vi "Config - resolve.vi"(8 "error in (no error)":errorcluster) -> (0 "error out":errorcluster)   [LabVIEW 2026, in "Tests.lvlib"]
doc: "Unit test (Caraya) for launch-config resolution.\nWith no config path the effective config equals the baseline inputs; a defined-but-missing path returns a non-fatal warning and falls back to the baseline; a present-but-invalid file (unparseable or schema-invalid) fails launch with no fallback.\nThe no-path and missing-path cases need no file; the invalid-file cases use a temp-root fixture that writes a malformed and a schema-invalid JSON file. Each expected error is captured and cleared per case.\n\nImplements LMBR-T-020, T-022, T-023 -> SRS-044, SRS-047, SRS-048. Assert-level IDs: Test-ID-Assert-Checklist.md."
uses:
  Tests.lvlib
  <vilib>/addons/_JKI Toolkits/Caraya/classes/Test/Test.lvclass
  <vilib>/addons/_JKI Toolkits/Caraya/classes/Assert/Assert.lvclass
  <vilib>/addons/_JKI Toolkits/Caraya/classes/Assert/Assert Equal Value_Variant.vi
  src/Lumberjack.lvlib
  src/TypeDefs/Severity.ctl
  src/TypeDefs/FilterMode.ctl
  src/TypeDefs/Filter.ctl
  src/TypeDefs/DropPolicy.ctl
  src/TypeDefs/AppenderConfig.ctl
  src/TypeDefs/FileConfig.ctl
  src/TypeDefs/FileAppenderConfig.ctl
  <vilib>/addons/_JKI Toolkits/Caraya/classes/Assert/Assert Error.vi
  <vilib>/addons/_JKI Toolkits/Caraya/classes/Assert/Assert False.vi
  <vilib>/addons/_JKI Toolkits/Caraya/classes/Assert/Assert True.vi
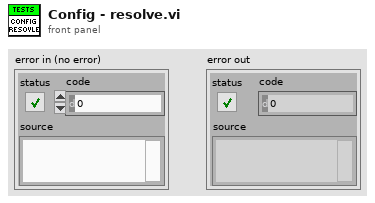
[diagram p1: front panel]
types:
  T1 = typedef "Lumberjack.lvlib/Severity.ctl" = enum16{"OFF", "FATAL", "ERROR", "WARN", "INFO", "DEBUG", "TRACE", "ALL"}
  T2 = typedef "Lumberjack.lvlib/FileAppenderConfig.ctl" = cluster{"common":T3, "file":T7}
  T3 = typedef "Lumberjack.lvlib/AppenderConfig.ctl" = cluster{"id":string, "threshold":T1, "filter":T4, "queueBound":i32, "dropPolicy":T6, "useUTC":bool}
  T4 = typedef "Lumberjack.lvlib/Filter.ctl" = cluster{"mode":T5, "levelMin":T1, "levelMax":T1, "tagPrefix":string}
  T5 = typedef "Lumberjack.lvlib/FilterMode.ctl" = enum16{"Mirror", "Routed"}
  T6 = typedef "Lumberjack.lvlib/DropPolicy.ctl" = enum16{"DropOldest", "DropNewest", "LevelAware"}
  T7 = typedef "Lumberjack.lvlib/FileConfig.ctl" = cluster{"rootFolder":path, "maxFileSize":i64, "maxFileCount":i32, "baseName":string, "extension":string, "delimiter":string, "calendarFolderTree":bool}
  T8 = typedef "Lumberjack.lvlib/LumberjackConfig.ctl" = cluster{"schemaVersion":string, "globalThreshold":T1, "defaultFileAppender":T2}
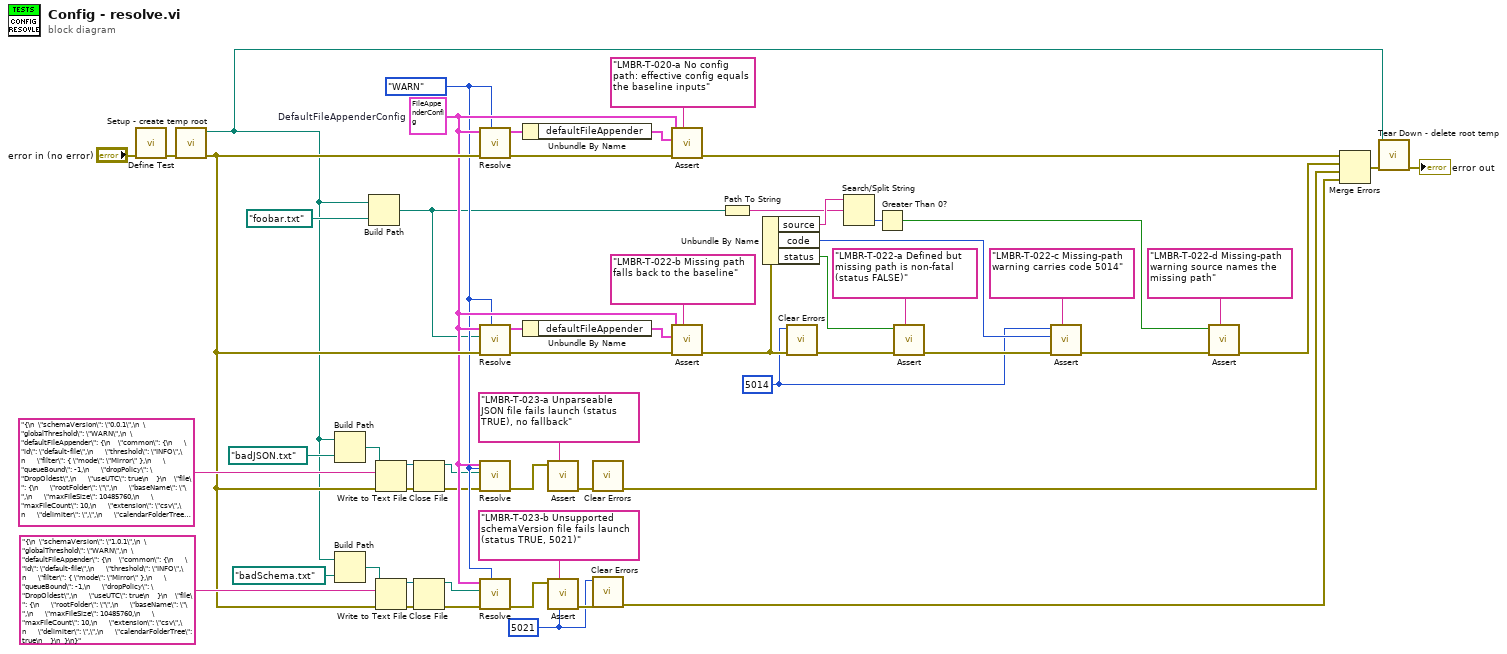
[diagram p0: block diagram]
diagram:
  w12 = 5014 ("error code (1)")
  w32 = 5021 ("error code (1)")
  w36 = Severity."WARN" ("GlobalThreshold")
  w37 = T2 {"common"={"id"="cfg-test", "threshold"=enum."ERROR", "filter"={"mode"=enum."Mirror", "levelMin"=enum."INFO", "levelMax"=enum."INFO", "tagPrefix"=""}, "queueBound"=250, "dropPolicy"=enum."DropNewest", "useUTC"=FALSE}, "file"={"rootFolder"=path "c:/Logs/cfgtest", "maxFileSize"=2097152, "maxFileCount"=7, "baseName"="cfg", "extension"="log", "delimiter"=";", "calendarFolderTree"=FALSE}}  # DefaultFileAppenderConfig
  n1 = call <vilib>:"Define Test.vi"("error in (no error)"="error in (no error)") -> ("error out"=w46:errorcluster)  [unwired: 9 in, 1 out]
  n2 = call "Setup - create temp root.vi"("error in (no error)"=w46) -> ("error out"=w38:errorcluster, "tempRoot"=w26:path)  [unwired: 9 in]
  n3 = Build Path(base path=w26, name or relative path=path "badJSON.txt") -> (appended path=w43:path)
  n4 = Build Path(base path=w26, name or relative path=path "badSchema.txt") -> (appended path=w39:path)
  n5 = Build Path(base path=w26, name or relative path=path "foobar.txt") -> (appended path=w20:path)
  n6 = Write to Text File(file (use dialog)=w43, text="{\n  \"schemaVersion\": \"0.0.1\",\n  \"globalThreshold\": \"WARN\",\n  \"defaultFileAppender\": {\n    \"common\": {\n      \"id\": \"default-file\",\n      \"threshold\": \"INFO\",\n      \"filter\": { \"mode\": \"Mirror\" },\n      \"queueBound\": -1,\n      \"dropPolicy\": \"DropOldest\",\n      \"useUTC\": true\n    }\n    \"file\": {\n      \"rootFolder\": \"\",\n      \"baseName\": \"\",\n      \"maxFileSize\": 10485760,\n      \"maxFileCount\": 10,\n      \"extension\": \"csv\",\n      \"delimiter\": \",\",\n      \"calendarFolderTree\": true\n    }\n  }\n}", error in=w38) -> (refnum out=w8:refnum<file>, error out=w4:errorcluster)  [unwired: 1 in, 1 out]
  n7 = Write to Text File(file (use dialog)=w39, text="{\n  \"schemaVersion\": \"1.0.1\",\n  \"globalThreshold\": \"WARN\",\n  \"defaultFileAppender\": {\n    \"common\": {\n      \"id\": \"default-file\",\n      \"threshold\": \"INFO\",\n      \"filter\": { \"mode\": \"Mirror\" },\n      \"queueBound\": -1,\n      \"dropPolicy\": \"DropOldest\",\n      \"useUTC\": true\n    }\n    \"file\": {\n      \"rootFolder\": \"\",\n      \"baseName\": \"\",\n      \"maxFileSize\": 10485760,\n      \"maxFileCount\": 10,\n      \"extension\": \"csv\",\n      \"delimiter\": \",\",\n      \"calendarFolderTree\": true\n    }\n  }\n}", error in=w38) -> (refnum out=w7:refnum<file>, error out=w6:errorcluster)  [unwired: 1 in, 1 out]
  n8 = Close File(refnum=w8, error in=w4) -> (path=w2:path, error out=w3:errorcluster)
  n9 = Close File(refnum=w7, error in=w6) -> (path=w1:path, error out=w5:errorcluster)
  n10 = call "Resolve.vi"("GlobalThreshold"=w36, "error in (no error)"=w38, "DefaultFileAppenderConfig"=w37) -> ("error out"=w55:errorcluster, "ResolvedConfig"=w53:T8)  [unwired: 7 in]
  n11 = call "Resolve.vi"("GlobalThreshold"=w36, "error in (no error)"=w38, "ConfigFilePath"=w20, "DefaultFileAppenderConfig"=w37) -> ("error out"=w47:errorcluster, "ResolvedConfig"=w48:T8)  [unwired: 6 in]
  n12 = call "Resolve.vi"("GlobalThreshold"=w36, "error in (no error)"=w3, "ConfigFilePath"=w2, "DefaultFileAppenderConfig"=w37) -> ("error out"=w35:errorcluster)  [unwired: 6 in, 1 out]
  n13 = call "Resolve.vi"("GlobalThreshold"=w36, "error in (no error)"=w5, "ConfigFilePath"=w1, "DefaultFileAppenderConfig"=w37) -> ("error out"=w34:errorcluster)  [unwired: 6 in, 1 out]
  n14 = Unbundle By Name(w53) -> ("defaultFileAppender"=w52:T2)
  n15 = Unbundle By Name(w48) -> ("defaultFileAppender"=w49:T2)
  n16 = call-poly <vilib>:"Assert.vi"("Label"="LMBR-T-023-a Unparseable JSON file fails launch (status TRUE), no fallback", "Error?"=w35) -> ("error out"=w25:errorcluster)  [unwired: 8 in, 1 out]
  n17 = call-poly <vilib>:"Assert.vi"("error code (1)"=w32, "Label"="LMBR-T-023-b Unsupported schemaVersion file fails launch (status TRUE, 5021)", "Error?"=w34) -> ("error out"=w33:errorcluster)  [unwired: 7 in, 1 out]
  n18 = call <vilib>:"Clear Errors.vi"("error in (no error)"=w25) -> ("error out"=w24:errorcluster)  [unwired: 5 in, 1 out]
  n19 = call <vilib>:"Clear Errors.vi"("error in (no error)"=w33, "specific error code to clear (0: all)"=w32) -> ("error out"=w28:errorcluster)  [unwired: 4 in, 1 out]
  n20 = call-poly <vilib>:"Assert.vi"("Label"="LMBR-T-020-a No config path: effective config equals the baseline inputs", "error in (no error)"=w55, "Actual"=w52, "Expected"=w37) -> ("error out"=w54:errorcluster)  [unwired: 6 in, 1 out]
  n21 = call-poly <vilib>:"Assert.vi"("Label"="LMBR-T-022-b Missing path falls back to the baseline", "error in (no error)"=w47, "Actual"=w49, "Expected"=w37) -> ("error out"=w14:errorcluster)  [unwired: 6 in, 1 out]
  n22 = Path To String(path=w20) -> (string=w9:string)
  n23 = Unbundle By Name(w14) -> ("source"=w10:string, "code"=w18:i32, "status"=w16:bool)
  n24 = call <vilib>:"Clear Errors.vi"("error in (no error)"=w14, "specific error code to clear (0: all)"=w12) -> ("error out"=w13:errorcluster)  [unwired: 4 in, 1 out]
  n25 = Search/Split String(string=w10, search string/char (-)=w9) -> (offset of match=w11:i32)  [unwired: 1 in, 2 out]
  n26 = Greater Than 0?(x=w11) -> (x > 0?=w15:bool)
  n27 = call-poly <vilib>:"Assert.vi"("Label"="LMBR-T-022-a Defined but missing path is non-fatal (status FALSE)", "error in (no error)"=w13, "False?"=w16) -> ("error out"=w17:errorcluster)  [unwired: 7 in, 1 out]
  n28 = call-poly <vilib>:"Assert.vi"("Label"="LMBR-T-022-c Missing-path warning carries code 5014", "error in (no error)"=w17, "Actual"=w18, "Expected"=w12) -> ("error out"=w22:errorcluster)  [unwired: 6 in, 1 out]
  n29 = call-poly <vilib>:"Assert.vi"("Label"="LMBR-T-022-d Missing-path warning source names the missing path", "error in (no error)"=w22, "True?"=w15) -> ("error out"=w21:errorcluster)  [unwired: 7 in, 1 out]
  n30 = Merge Errors(w54, w21, w24, w28) -> (w29:errorcluster)
  n31 = call "Tear Down - delete root temp.vi"("error in (no error)"=w29, "tempRoot"=w26) -> ("error out"=→"error out":errorcluster)  [unwired: 9 in]
